vi "VI Tree.vi"   [LabVIEW 2016, in "BK Precision 9200 Series.lvlib"]
doc: "This is the instrument driver for the B&K Precision 9200 series DC power supplies. The VI Tree displays all the user-callable VIs of the instrument driver in an organized table."
uses:
  <instrlib>/BK Precision 9200 Series/BK Precision 9200 Series.lvlib
panel:
  # "(c) 2014 B&K Precision Corporation.  ALL RIGHTS RESERVED."
  # "SEE DIAGRAM\nFOR VI TREE."
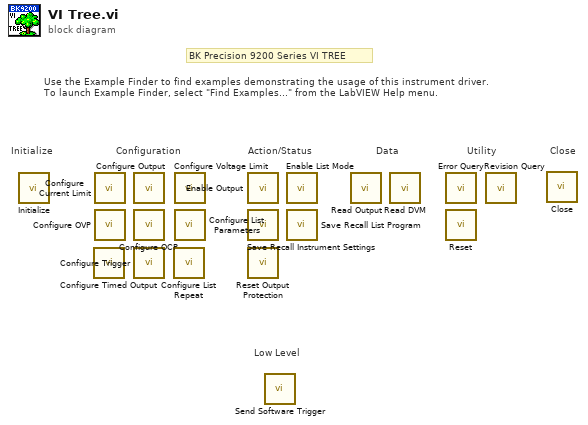
[diagram p0: block diagram]
diagram:
  # "Low Level"
  # "BK Precision 9200 Series VI TREE"
  # "Use the Example Finder to find examples demonstrating the usage of this instrument driver.\nTo launch Example Finder, select \"Find Examples...\" from the LabVIEW Help menu."
  # "Configuration"
  # "Utility"
  # "Data"
  # "Action/Status"
  # "Close"
  # "Initialize"
  n1 = call <instrlib>:"Initialize.vi"() -> ()  [unwired: 10 in, 2 out]
  n2 = call <instrlib>:"Configure Timed Output.vi"() -> ()  [unwired: 10 in, 2 out]
  n3 = call <instrlib>:"Configure Current Limit.vi"() -> ()  [unwired: 10 in, 2 out]
  n4 = call <instrlib>:"Configure OVP.vi"() -> ()  [unwired: 10 in, 2 out]
  n5 = call <instrlib>:"Configure Output.vi"() -> ()  [unwired: 10 in, 2 out]
  n6 = call <instrlib>:"Configure OCP.vi"() -> ()  [unwired: 10 in, 2 out]
  n7 = call <instrlib>:"Configure Trigger.vi"() -> ()  [unwired: 10 in, 2 out]
  n8 = call <instrlib>:"Configure List Repeat.vi"() -> ()  [unwired: 10 in, 2 out]
  n9 = call <instrlib>:"Configure Voltage Limit.vi"() -> ()  [unwired: 10 in, 2 out]
  n10 = call <instrlib>:"Configure List Parameters.vi"() -> ()  [unwired: 14 in, 2 out]
  n11 = call <instrlib>:"Enable Output.vi"() -> ()  [unwired: 10 in, 2 out]
  n12 = call <instrlib>:"Save Recall Instrument Settings.vi"() -> ()  [unwired: 10 in, 2 out]
  n13 = call <instrlib>:"Reset Output Protection.vi"() -> ()  [unwired: 10 in, 2 out]
  n14 = call <instrlib>:"Send Software Trigger.vi"() -> ()  [unwired: 10 in, 2 out]
  n15 = call <instrlib>:"Enable List Mode.vi"() -> ()  [unwired: 10 in, 2 out]
  n16 = call <instrlib>:"Save Recall List Program.vi"() -> ()  [unwired: 10 in, 2 out]
  n17 = call <instrlib>:"Read Output.vi"() -> ()  [unwired: 11 in, 5 out]
  n18 = call <instrlib>:"Read DVM.vi"() -> ()  [unwired: 9 in, 3 out]
  n19 = call <instrlib>:"Error Query.vi"() -> ()  [unwired: 8 in, 4 out]
  n20 = call <instrlib>:"Reset.vi"() -> ()  [unwired: 10 in, 2 out]
  n21 = call <instrlib>:"Revision Query.vi"() -> ()  [unwired: 8 in, 4 out]
  n22 = call <instrlib>:"Close.vi"() -> ()  [unwired: 11 in, 1 out]
